vi "Stop Core.vi"(10 "final error code":i32, 11 "IViewModel in":refnum<class "IViewModel.lvclass">) -> (3 "IViewModel out":refnum<class "IViewModel.lvclass">)   [LabVIEW 2015, in "IViewModel.lvlib" / "IViewModel.lvclass"]
doc: "(<B>Filename</B>: Actor Framework.lvlib:Actor.lvclass:Stop Core.vi)\n\nDefines what the actor does before it stops. Use the <B>final error code</B> input to determine whether the actor shut down in response to an error.\n\nBy default, this method does nothing. A descendant class may override it to define behavior, such as shutting down any processes the actor initiated in its override of the Actor Core method.\n\n<License>\nCopyright © 2017 Composed Systems, LLC | All rights reserved\nwww.composed.io\n\nAuthor: Ethan Stern <ethan.stern@composed.io>\n\nThis software is provided \"AS IS\" WITHOUT WARRANTIES, either express or implied, AND IS FOR EDUCATIONAL PURPOSES ONLY.\n</License>"
uses:
  IViewModel.lvclass
  IViewModel.lvclass/IViewModel.ctl
  <vilib>/ActorFramework/Message Enqueuer/Message Enqueuer.lvclass/Message Enqueuer.ctl
  <vilib>/ActorFramework/Message Enqueuer/Enqueue.vi
  <vilib>/ActorFramework/Message Priority Queue/Priority Enqueue.vi
  IViewManager/IViewManager/IViewManager.lvclass
  <vilib>/ActorFramework/Stop Msg/Stop Msg.lvclass
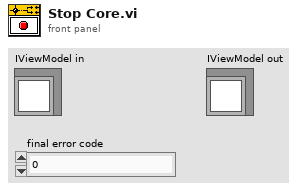
[diagram p1: front panel]
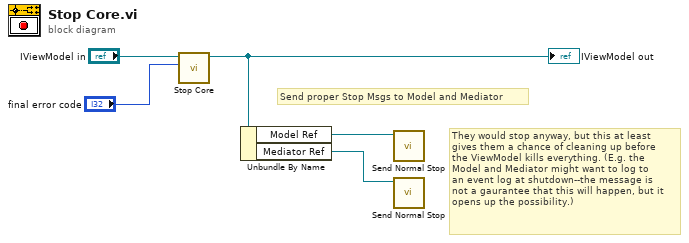
[diagram p0: block diagram]
diagram:
  # "Send proper Stop Msgs to Model and Mediator"
  # "They would stop anyway, but this at least\ngives them a chance of cleaning up before\nthe ViewModel kills everything. (E.g. the\nModel and Mediator might want to log to\nan event log at shutdown--the message is\nnot a gaurantee that this will happen, but it\nopens up the possibility.)"
  n1 = call-parent "Stop Core.vi"("final error code"="final error code", "IViewable in"="IViewModel in") -> ("IViewable out"=w3:refnum<class "IViewModel.lvclass">)  [unwired: 9 in]
  "IViewModel out" <- w3
  n2 = Unbundle By Name(w3) -> ("Model Ref"=w2:refnum<class "Message Enqueuer.lvclass">, "Mediator Ref"=w1:refnum<class "Message Enqueuer.lvclass">)
  n3 = call <vilib>:"Send Normal Stop.vi"("Message Enqueuer"=w2) -> ()  [unwired: 10 in, 1 out]
  n4 = call <vilib>:"Send Normal Stop.vi"("Message Enqueuer"=w1) -> ()  [unwired: 10 in, 1 out]
